vi "USERPRODUCER.vi"() -> ()   [LabVIEW 2024]
doc: "Use this template to build a producer/consumer design pattern. Use this template when you need to execute a process, such as data analysis, when a data source, such as a triggered acquisition, produces data at an uneven rate and you need to execute the process when the data becomes available."
uses:
  <vilib>/DAQmx/read.llb/DAQmx Read (Analog 2D DBL NChan NSamp).vi
  <vilib>/DAQmx/miscellaneous.llb/DAQmx Fill In Error Info.vi
  <vilib>/Utility/TDMS File Viewer/NI_TDMS File Viewer.lvlib
panel:
  out "data":dbl[][](array[numeric]) format="%0.2f"
  out "error out":errorcluster
  in  "file path":path
  in  "operation (0:open)":T1(ring)
  in  "file format version (2.0)":enum16{"1.0", "2.0"}(ring)
  out "2D DBL":dbl[][](graph) caption="data"
  in  "STOP":bool caption="stop"
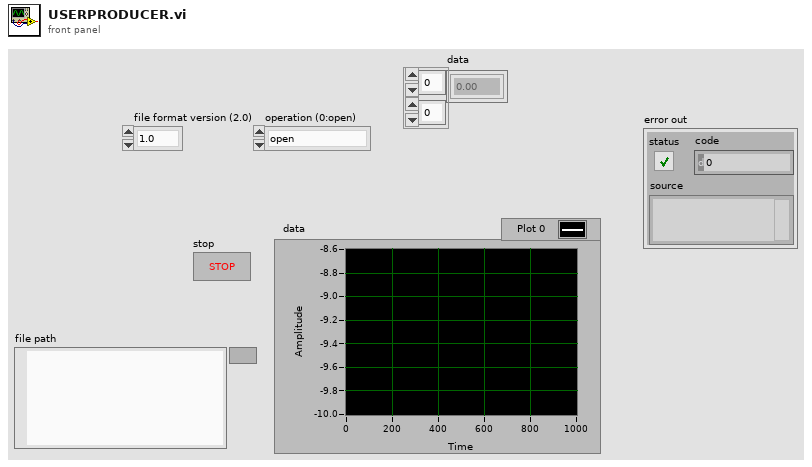
[diagram p1: front panel]
types:
  T1 = enum16{"open", "open or create", "create or replace", "create", "open (read-only)"}
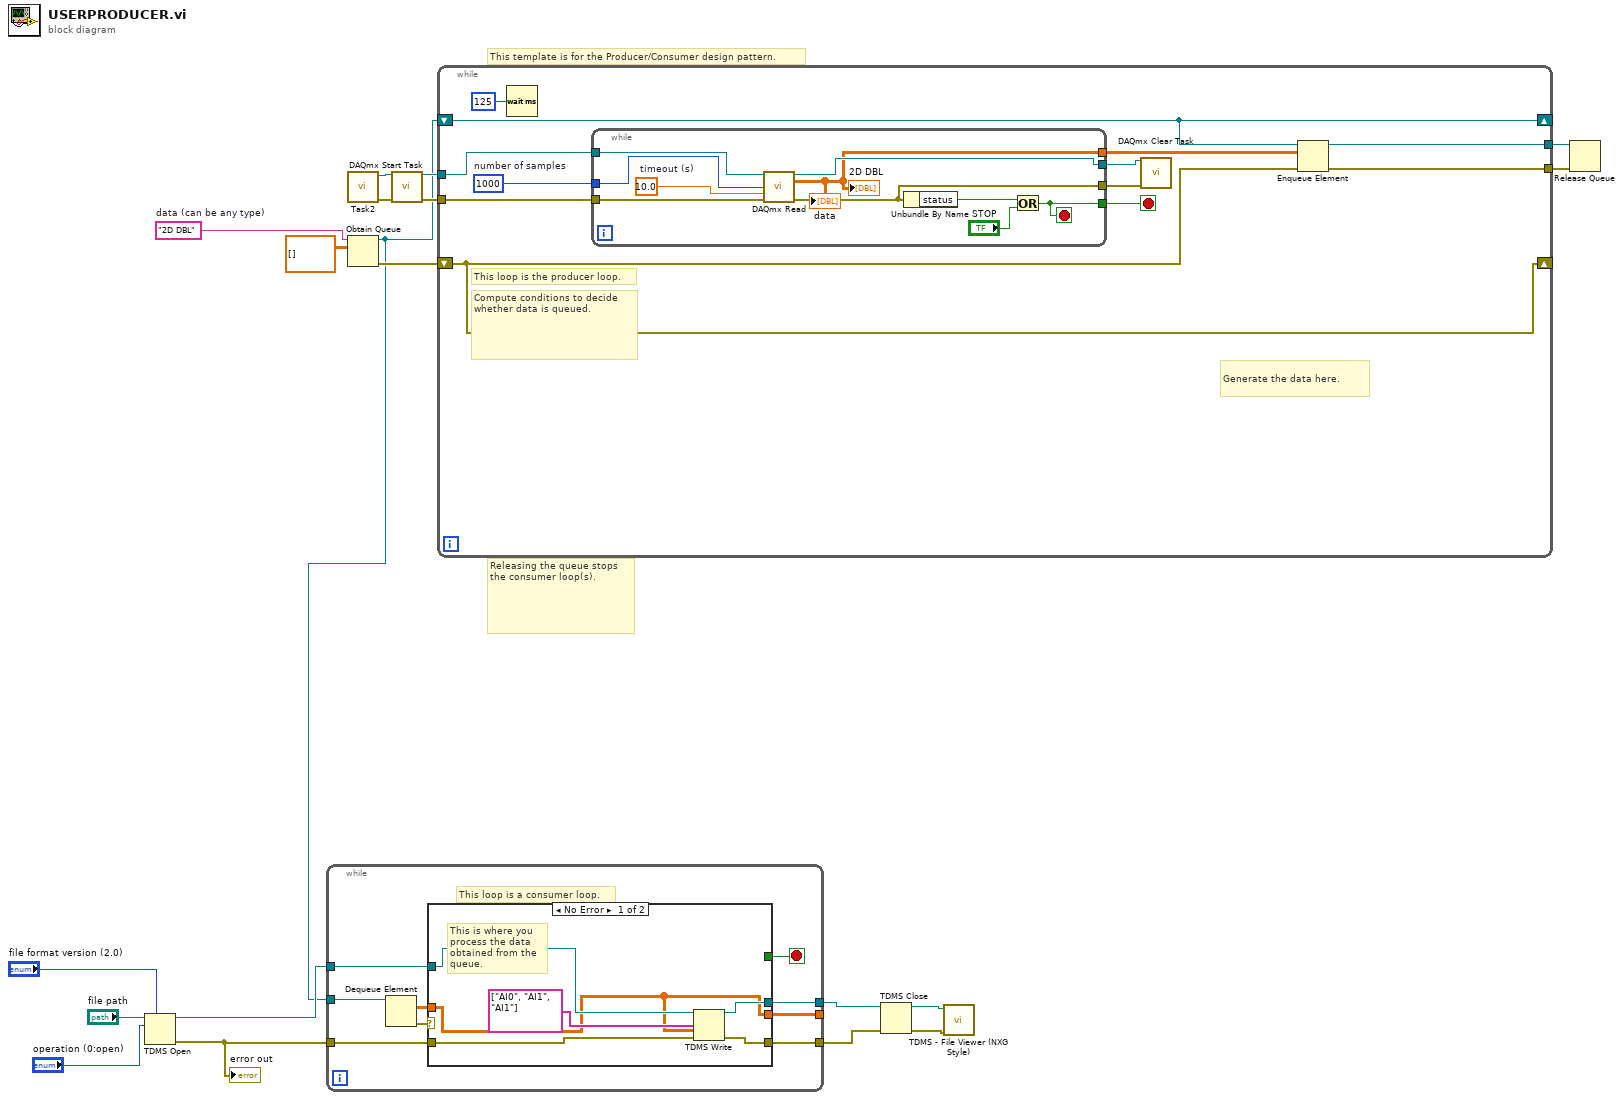
[diagram p0: block diagram]
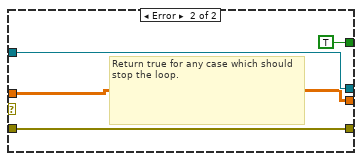
[diagram p2: hidden frame]
diagram:
  w14 = "2D DBL"  # data (can be any type)
  # "Releasing the queue stops the consumer loop(s)."
  # "This template is for the Producer/Consumer design pattern."
  n1 = TDMS Open(7:"file format version (2.0)", 10:"operation (0:open)", 11:"file path") -> (0:w8:errorcluster, 3:w7:refnum<k34>)  [unwired: 4 in]
  "error out" <- w8
  n2 = call "Task2.vi"() -> ("error out"=w15:errorcluster, "task out"=w16:refnum<k21>)  [unwired: 10 in]
  n3 = Obtain Queue(name (unnamed)=w14, element data type=dbl[][] []) -> (queue out=w6:refnum<queue>, error out=w19:errorcluster)  [unwired: 3 in, 1 out]
  n4 = while {
    tunnel: w6 -> [w28]
    tunnel: w8 -> [w24]
    tunnel: w7 -> [w23]
    tunnel: [w22] -> w4
    tunnel: [w21] -> w3
    tunnel: [w20] -> _
    stop <- w25 stop-if-true
    # "This loop is a consumer loop."
    n5 = Dequeue Element(queue=w28) -> (element=w26:dbl[][], error out=w27:errorcluster)  [unwired: 2 in, 2 out]
    n6 = case shown="No Error" w27 {
      tunnel: w26 -> [w29 w35]
      tunnel: [_ TRUE] -> w25
      tunnel: w24 -> [w34 w37]
      tunnel: w23 -> [w33 w36]
      tunnel: [w32 w36] -> w22
      tunnel: [w31 w37] -> w21
      tunnel: [w29 w35] -> w20
      frame No Error {
        # "This is where you process the data obtained from the queue."
        n7 = TDMS Write(0:w33, 7:string[] ["AI0", "AI1", "AI1"] ("channel name(s) in (Untitled)"), 9:w29, 11:w34) -> (4:w32:refnum<k34>, 15:w31:errorcluster)  [unwired: 2 in, 2 out]
      }
      frame Error {
        # "Return true for any case which should stop the loop."
      }
    }
  }
  n8 = call <vilib>:"DAQmx Start Task.vi"("task/channels in"=w16, "error in"=w15) -> ("task out"=w18:refnum<k21>, "error out"=w17:errorcluster)  [unwired: 12 in]
  n9 = while {
    shift-right: [w43] -> _
    shift-left: w19 -> [w43]
    shift-right: [w39] -> _
    shift-left: w6 -> [w39]
    tunnel: w18 -> [w49]
    tunnel: w17 -> [w47]
    tunnel: [w41] -> w10
    tunnel: [w40] -> w9
    stop <- w42 stop-if-true
    w48 = 1000  # number of samples
    # "Generate the data here."
    # "Compute conditions to decide whether data is queued."
    # "This loop is the producer loop."
    n10 = Wait (ms)(milliseconds to wait=u32 125) -> ()  [unwired: 1 out]
    n11 = while {
      tunnel: w49 -> [w58]
      tunnel: w48 -> [w57]
      tunnel: w47 -> [w55]
      tunnel: [w54] -> w46
      tunnel: [w52] -> w45
      tunnel: [w53] -> w44
      tunnel: [w51] -> w42
      stop <- w51 stop-if-true
      w56 = 10.0  # timeout (s)
      n12 = call-poly <vilib>:"DAQmx Read.vi"("task/channels in"=w58, "number of samples per channel"=w57, "timeout"=w56, "error in"=w55) -> ("task out"=w54:refnum<k21>, "data"=w52:dbl[][], "error out"=w53:errorcluster)  [unwired: 9 in]
      "2D DBL" <- w52
      "data" <- w52
      n13 = Unbundle By Name(w53) -> ("status"=w59:bool)
      n14 = Or(x=w59, y="STOP") -> (x .or. y?=w51:bool)
    }
    n15 = call <vilib>:"DAQmx Clear Task.vi"("task in"=w46, "error in"=w44) -> ()  [unwired: 13 in, 1 out]
    n16 = Enqueue Element(queue=w39, element=w45, error in (no error)=w43) -> (queue out=w41:refnum<queue>, error out=w40:errorcluster)  [unwired: 1 in, 1 out]
  }
  n17 = TDMS Close(8:w3, 11:w4) -> (0:w1:errorcluster, 3:w2:path)
  n18 = call <vilib>:"TDMS - File Viewer (NXG Style).vi"("error in"=w1, "file in"=w2) -> ()  [unwired: 8 in, 2 out]
  n19 = Release Queue(queue=w10, error in (no error)=w9) -> ()  [unwired: 1 in, 3 out]
